vi "Read Raw.vi"(6 "Maximum Time (10000 ms)":u32=10000, 8 "error in (no error)":errorcluster, 9 "Select Trace (1: 1)":u16(ring)=1 items=["1"=1, "2"=2, "3"=3, "4"=4, "5"=5, "6"=6, "7"=7, "8"=8], 10 "Measurement Type (6: Phase Noise)":u16(ring)=6 items=["AM Noise"=1, "Baseband Noise"=2, "Freq/Power"=3, "Spectrum"=4, "Transient"=5, "Phase Noise"=6, "User"=7], 11 "VISA resource name":refnum<visa-resource-name>) -> (0 "error out":errorcluster, 2 "Measurements":dbl[](array[numeric]) format="%^#_9g", 3 "VISA resource name out":refnum<visa-resource-name>)   [LabVIEW 2011, in "Agilent E5052X.lvlib"]
doc: "Reads Raw trace data from the instrument."
uses:
  Agilent E5052X.lvlib
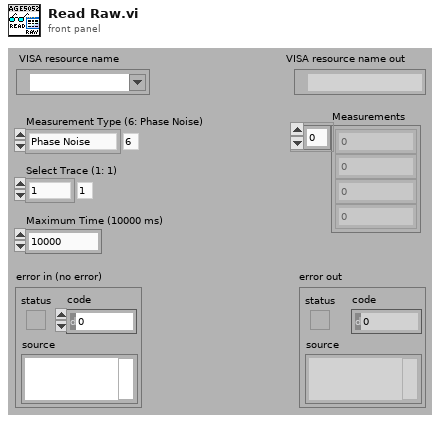
[diagram p1: front panel]
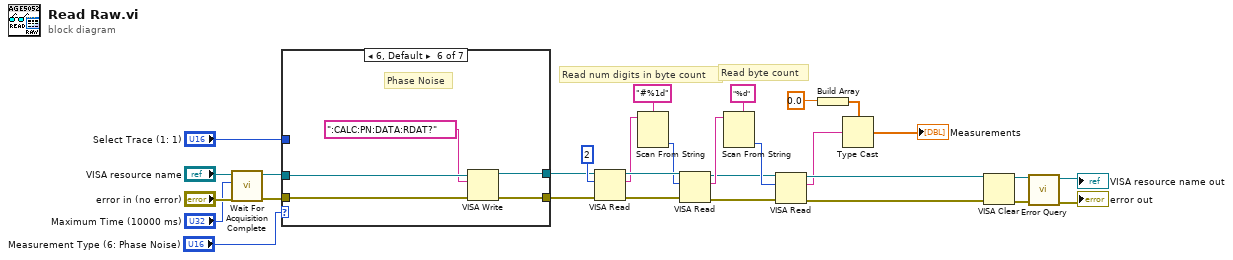
[diagram p0: block diagram]
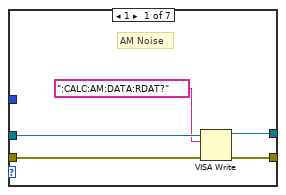
[diagram p2: hidden frame]
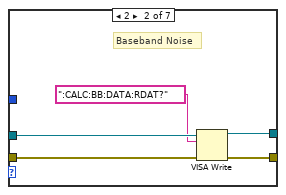
[diagram p3: hidden frame]
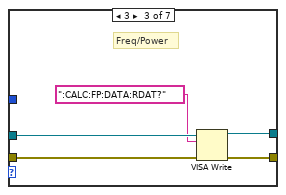
[diagram p4: hidden frame]
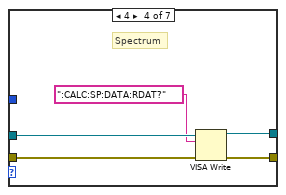
[diagram p5: hidden frame]
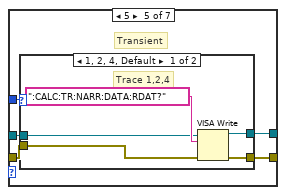
[diagram p6: hidden frame]
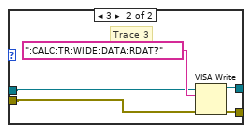
[diagram p7: hidden frame]
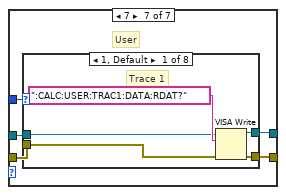
[diagram p8: hidden frame]
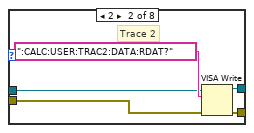
[diagram p9: hidden frame]
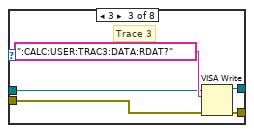
[diagram p10: hidden frame]
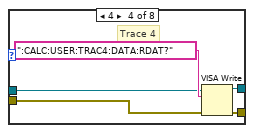
[diagram p11: hidden frame]
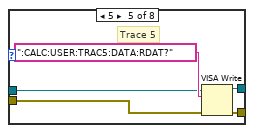
[diagram p12: hidden frame]
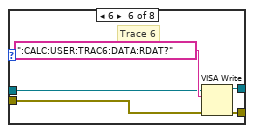
[diagram p13: hidden frame]
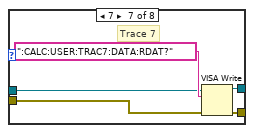
[diagram p14: hidden frame]
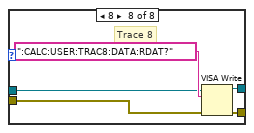
[diagram p15: hidden frame]
diagram:
  # "Read num digits in byte count"
  # "Read byte count"
  n1 = call "Wait For Acquisition Complete.vi"("error in (no error)"="error in (no error)", "Maximum Time (10000)"="Maximum Time (10000 ms)", "VISA resource name"="VISA resource name") -> ("error out"=w10:errorcluster, "VISA resource name out"=w11:refnum<visa-resource-name>)  [unwired: 7 in]
  n2 = case shown="6, Default" "Measurement Type (6: Phase Noise)" {
    tunnel: w11 -> [w35 w40 w45 w50 w55 w70 w74]
    tunnel: w10 -> [w34 w39 w44 w49 w54 w69 w73]
    tunnel: "Select Trace (1: 1)" -> [_ _ _ _ w51 _ w75]
    tunnel: [w33 w38 w43 w48 w53 w68 w72] -> w19
    tunnel: [w32 w37 w42 w47 w52 w67 w71] -> w18
    frame 1 {
      # "AM Noise"
      n3 = VISA Write(VISA resource name=w35, write buffer=":CALC:AM:DATA:RDAT?" ("format string"), error in (no error)=w34) -> (VISA resource name out=w33:refnum<visa-resource-name>, error out=w32:errorcluster)  [unwired: 1 out]
    }
    frame 2 {
      # "Baseband Noise"
      n4 = VISA Write(VISA resource name=w40, write buffer=":CALC:BB:DATA:RDAT?" ("format string"), error in (no error)=w39) -> (VISA resource name out=w38:refnum<visa-resource-name>, error out=w37:errorcluster)  [unwired: 1 out]
    }
    frame 3 {
      # "Freq/Power"
      n5 = VISA Write(VISA resource name=w45, write buffer=":CALC:FP:DATA:RDAT?" ("format string"), error in (no error)=w44) -> (VISA resource name out=w43:refnum<visa-resource-name>, error out=w42:errorcluster)  [unwired: 1 out]
    }
    frame 4 {
      # "Spectrum"
      n6 = VISA Write(VISA resource name=w50, write buffer=":CALC:SP:DATA:RDAT?" ("format string"), error in (no error)=w49) -> (VISA resource name out=w48:refnum<visa-resource-name>, error out=w47:errorcluster)  [unwired: 1 out]
    }
    frame 5 {
      # "Transient"
      n7 = case shown="1, 2, 4, Default" w51 {
        tunnel: w55 -> [w59 w64]
        tunnel: w54 -> [w58 w63]
        tunnel: [w57 w62] -> w53
        tunnel: [w56 w61] -> w52
        frame 1, 2, 4, Default {
          # "Trace 1,2,4"
          n8 = VISA Write(VISA resource name=w59, write buffer=":CALC:TR:NARR:DATA:RDAT?" ("format string"), error in (no error)=w58) -> (VISA resource name out=w57:refnum<visa-resource-name>, error out=w56:errorcluster)  [unwired: 1 out]
        }
        frame 3 {
          # "Trace 3"
          n9 = VISA Write(VISA resource name=w64, write buffer=":CALC:TR:WIDE:DATA:RDAT?" ("format string"), error in (no error)=w63) -> (VISA resource name out=w62:refnum<visa-resource-name>, error out=w61:errorcluster)  [unwired: 1 out]
        }
      }
    }
    frame 6, Default {
      # "Phase Noise"
      n10 = VISA Write(VISA resource name=w70, write buffer=":CALC:PN:DATA:RDAT?" ("format string"), error in (no error)=w69) -> (VISA resource name out=w68:refnum<visa-resource-name>, error out=w67:errorcluster)  [unwired: 1 out]
    }
    frame 7 {
      # "User"
      n11 = case shown="1, Default" w75 {
        tunnel: w74 -> [w79 w84 w89 w94 w99 w104 w109 w114]
        tunnel: w73 -> [w78 w83 w88 w93 w98 w103 w108 w113]
        tunnel: [w77 w82 w87 w92 w97 w102 w107 w112] -> w72
        tunnel: [w76 w81 w86 w91 w96 w101 w106 w111] -> w71
        frame 1, Default {
          # "Trace 1"
          n12 = VISA Write(VISA resource name=w79, write buffer=":CALC:USER:TRAC1:DATA:RDAT?" ("format string"), error in (no error)=w78) -> (VISA resource name out=w77:refnum<visa-resource-name>, error out=w76:errorcluster)  [unwired: 1 out]
        }
        frame 2 {
          # "Trace 2"
          n13 = VISA Write(VISA resource name=w84, write buffer=":CALC:USER:TRAC2:DATA:RDAT?" ("format string"), error in (no error)=w83) -> (VISA resource name out=w82:refnum<visa-resource-name>, error out=w81:errorcluster)  [unwired: 1 out]
        }
        frame 3 {
          # "Trace 3"
          n14 = VISA Write(VISA resource name=w89, write buffer=":CALC:USER:TRAC3:DATA:RDAT?" ("format string"), error in (no error)=w88) -> (VISA resource name out=w87:refnum<visa-resource-name>, error out=w86:errorcluster)  [unwired: 1 out]
        }
        frame 4 {
          # "Trace 4"
          n15 = VISA Write(VISA resource name=w94, write buffer=":CALC:USER:TRAC4:DATA:RDAT?" ("format string"), error in (no error)=w93) -> (VISA resource name out=w92:refnum<visa-resource-name>, error out=w91:errorcluster)  [unwired: 1 out]
        }
        frame 5 {
          # "Trace 5"
          n16 = VISA Write(VISA resource name=w99, write buffer=":CALC:USER:TRAC5:DATA:RDAT?" ("format string"), error in (no error)=w98) -> (VISA resource name out=w97:refnum<visa-resource-name>, error out=w96:errorcluster)  [unwired: 1 out]
        }
        frame 6 {
          # "Trace 6"
          n17 = VISA Write(VISA resource name=w104, write buffer=":CALC:USER:TRAC6:DATA:RDAT?" ("format string"), error in (no error)=w103) -> (VISA resource name out=w102:refnum<visa-resource-name>, error out=w101:errorcluster)  [unwired: 1 out]
        }
        frame 7 {
          # "Trace 7"
          n18 = VISA Write(VISA resource name=w109, write buffer=":CALC:USER:TRAC7:DATA:RDAT?" ("format string"), error in (no error)=w108) -> (VISA resource name out=w107:refnum<visa-resource-name>, error out=w106:errorcluster)  [unwired: 1 out]
        }
        frame 8 {
          # "Trace 8"
          n19 = VISA Write(VISA resource name=w114, write buffer=":CALC:USER:TRAC8:DATA:RDAT?" ("format string"), error in (no error)=w113) -> (VISA resource name out=w112:refnum<visa-resource-name>, error out=w111:errorcluster)  [unwired: 1 out]
        }
      }
    }
  }
  n20 = VISA Read(VISA resource name=w19, byte count=u32 2, error in (no error)=w18) -> (VISA resource name out=w24:refnum<visa-resource-name>, read buffer=w20:string, error out=w25:errorcluster)  [unwired: 1 out]
  n21 = Scan From String(format string="#%1d", input string=w20) -> (output 1=w23:i32)  [unwired: 3 in, 3 out]
  n22 = VISA Read(VISA resource name=w24, byte count=w23, error in (no error)=w25) -> (VISA resource name out=w16:refnum<visa-resource-name>, read buffer=w22:string, error out=w15:errorcluster)  [unwired: 1 out]
  n23 = Scan From String(format string="%d", input string=w22) -> (output 1=w17:i32)  [unwired: 3 in, 3 out]
  n24 = VISA Read(VISA resource name=w16, byte count=w17, error in (no error)=w15) -> (VISA resource name out=w13:refnum<visa-resource-name>, read buffer=w2:string, error out=w12:errorcluster)  [unwired: 1 out]
  n25 = Build Array(sgl 0.0) -> (w3:sgl[])
  n26 = Type Cast(type=w3, x=w2) -> (*(type *) &x=→"Measurements":sgl[])
  n27 = VISA Clear(VISA resource name=w13, error in (no error)=w12) -> (VISA resource name out=w7:refnum<visa-resource-name>, error out=w6:errorcluster)
  n28 = call "Error Query.vi"("error in (no error)"=w6, "VISA resource name"=w7) -> ("error out"=→"error out":errorcluster, "VISA resource name out"=→"VISA resource name out":refnum<visa-resource-name>)  [unwired: 6 in, 2 out]
